vi "setYrange.vi"(10 "name/data":string[][](array[string]), 11 "Array":refnum<vi>[](array[refnum])) -> (3 "element":string)   [LabVIEW 2013]
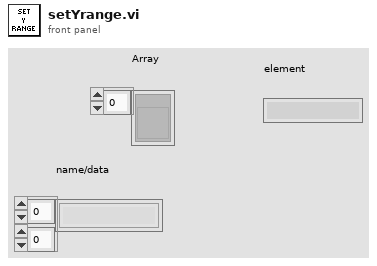
[diagram p1: front panel]
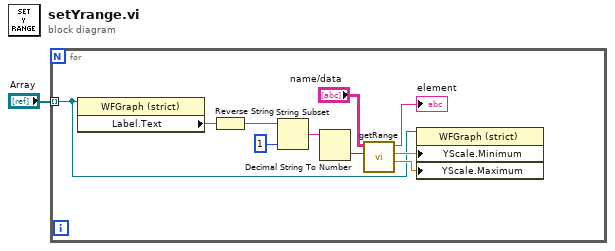
[diagram p0: block diagram]
diagram:
  n1 = for {
    tunnel: "Array" -> [w7] mode=indexing
    n2 = property class="WFGraph (strict)"(reference=w7) -> ("Label.Text"=w5:string)  [unwired: 1 in, 2 out]
    n3 = Reverse String(1:w5) -> (0:w4:string)
    n4 = String Subset(string=w4, length (rest)=1 ("length (rest)")) -> (substring=w3:string)  [unwired: 1 in]
    n5 = Decimal String To Number(string=w3) -> (number=w2:i32)  [unwired: 2 in, 1 out]
    n6 = call "getRange.vi"("channelNR"=w2, "name/data"="name/data") -> ("YMax"=w11:dbl, "YMin"=w10:dbl, "element"=→"element":string)  [unwired: 7 in]
    n7 = property class="WFGraph (strict)"(reference=w7, "YScale.Minimum"=w10, "YScale.Maximum"=w11) -> ()  [unwired: 1 in, 2 out]
  }
